vi "Clear.vi"(8 "error in (no error)":errorcluster, 11 "Process In":refnum<class "Mock Debug Message Receiver.lvclass">) -> (0 "error out":errorcluster)   [LabVIEW 2020, in "Mock Debug Message Receiver.lvclass"]
doc: "Clears any resorces allocated during initialization."
uses:
  Mock Debug Message Receiver.lvclass
  Mock Debug Message Receiver.lvclass/Mock Debug Message Receiver.ctl
  Process/Debug Process.lvclass
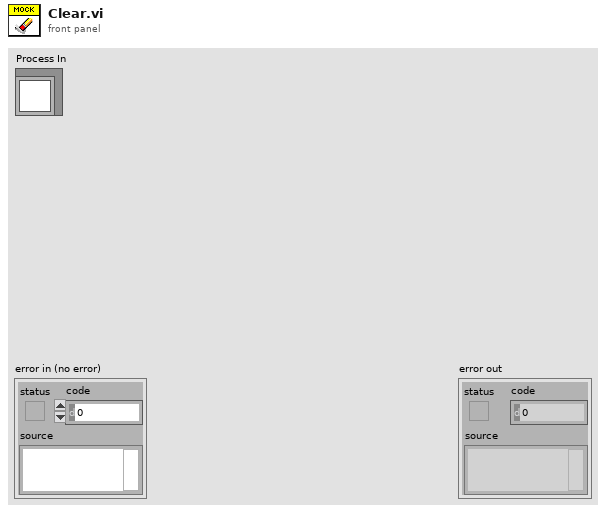
[diagram p1: front panel]
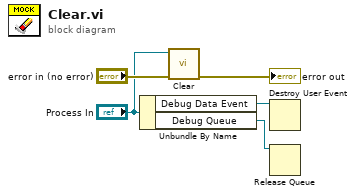
[diagram p0: block diagram]
diagram:
  n1 = Unbundle By Name("Process In") -> ("Debug Data Event"=w2:refnum<user-event>, "Debug Queue"=w1:refnum<queue>)
  n2 = call-parent "Clear.vi"("error in (no error)"="error in (no error)", "Process In"="Process In") -> ("error out"=→"error out":errorcluster)  [unwired: 9 in]
  n3 = Destroy User Event(user event=w2) -> ()  [unwired: 1 in, 1 out]
  n4 = Release Queue(queue=w1) -> ()  [unwired: 2 in, 3 out]
